vi "EVT Camera Open.vi"(10 "deviceInfo":T1, 11 "cameraHandle":u64) -> (1 "name":string, 2 "deviceInfo out":T1, 3 "cameraHandle out":u64, 4 "function return":u32(ring), 5 "fullName":string)   [LabVIEW 2019, in "EmergentCameraC.lvlib"]
doc: "EMERGENTCAMERAC_API EVT_ERROR EVT_CameraOpen(Camera_Handle* cameraHandle, struct GigEVisionDeviceInfo* deviceInfo);"
uses:
  <vilib>/Utility/importsl/GetValueByPointer/datatype.ctl
  <vilib>/Utility/importsl/GetValueByPointer/GetValueByPointer.xnode
  EmergentCameraC.lvlib
  emergentInstall_Windows/win64/eSDK/bin/EmergentCameraC.dll
types:
  T1 = cluster{"specVersionMajor":u16, "specVersionMinor":u16, "deviceMode":u32, "macAddress[0]":i8, "macAddress[1]":i8, "macAddress[2]":i8, "macAddress[3]":i8, "macAddress[4]":i8, "macAddress[5]":i8, "macAddress[6]":i8, "macAddress[7]":i8, "macAddress[8]":i8, "macAddress[9]":i8, "macAddress[10]":i8, "macAddress[11]":i8, "macAddress[12]":i8, "macAddress[13]":i8, "macAddress[14]":i8, "macAddress[15]":i8, "macAddress[16]":i8, "macAddress[17]":i8, "@dummy control@":i8, "@dummy control@":i8, "ipConfigOptions":u32, "ipConfigCurrent":u32, "currentIp[0]":i8, "currentIp[1]":i8, "currentIp[2]":i8, "currentIp[3]":i8, "currentIp[4]":i8, "currentIp[5]":i8, "currentIp[6]":i8, "currentIp[7]":i8, "currentIp[8]":i8, "currentIp[9]":i8, "currentIp[10]":i8, "currentIp[11]":i8, "currentIp[12]":i8, "currentIp[13]":i8, "currentIp[14]":i8, "currentIp[15]":i8, "currentSubnetMask[0]":i8, "currentSubnetMask[1]":i8, "currentSubnetMask[2]":i8, "currentSubnetMask[3]":i8, "currentSubnetMask[4]":i8, "currentSubnetMask[5]":i8, "currentSubnetMask[6]":i8, "currentSubnetMask[7]":i8, "currentSubnetMask[8]":i8, "currentSubnetMask[9]":i8, "currentSubnetMask[10]":i8, "currentSubnetMask[11]":i8, "currentSubnetMask[12]":i8, "currentSubnetMask[13]":i8, "currentSubnetMask[14]":i8, "currentSubnetMask[15]":i8, "defaultGateway[0]":i8, "defaultGateway[1]":i8, "defaultGateway[2]":i8, "defaultGateway[3]":i8, "defaultGateway[4]":i8, "defaultGateway[5]":i8, "defaultGateway[6]":i8, "defaultGateway[7]":i8, "defaultGateway[8]":i8, "defaultGateway[9]":i8, "defaultGateway[10]":i8, "defaultGateway[11]":i8, "defaultGateway[12]":i8, "defaultGateway[13]":i8, "defaultGateway[14]":i8, "defaultGateway[15]":i8, "manufacturerName[0]":i8, "manufacturerName[1]":i8, "manufacturerName[2]":i8, "manufacturerName[3]":i8, "manufacturerName[4]":i8, "manufacturerName[5]":i8, "manufacturerName[6]":i8, "manufacturerName[7]":i8, "manufacturerName[8]":i8, "manufacturerName[9]":i8, "manufacturerName[10]":i8, "manufacturerName[11]":i8, "manufacturerName[12]":i8, "manufacturerName[13]":i8, "manufacturerName[14]":i8, "manufacturerName[15]":i8, "manufacturerName[16]":i8, "manufacturerName[17]":i8, "manufacturerName[18]":i8, "manufacturerName[19]":i8, "manufacturerName[20]":i8, "manufacturerName[21]":i8, "manufacturerName[22]":i8, "manufacturerName[23]":i8, "manufacturerName[24]":i8, "manufacturerName[25]":i8, "manufacturerName[26]":i8, "manufacturerName[27]":i8, "manufacturerName[28]":i8, "manufacturerName[29]":i8, "manufacturerName[30]":i8, "manufacturerName[31]":i8, "modelName[0]":i8, "modelName[1]":i8, "modelName[2]":i8, "modelName[3]":i8, "modelName[4]":i8, "modelName[5]":i8, "modelName[6]":i8, "modelName[7]":i8, "modelName[8]":i8, "modelName[9]":i8, "modelName[10]":i8, "modelName[11]":i8, "modelName[12]":i8, "modelName[13]":i8, "modelName[14]":i8, "modelName[15]":i8, "modelName[16]":i8, "modelName[17]":i8, "modelName[18]":i8, "modelName[19]":i8, "modelName[20]":i8, "modelName[21]":i8, "modelName[22]":i8, "modelName[23]":i8, "modelName[24]":i8, "modelName[25]":i8, "modelName[26]":i8, "modelName[27]":i8, "modelName[28]":i8, "modelName[29]":i8, "modelName[30]":i8, "modelName[31]":i8, "deviceVersion[0]":i8, "deviceVersion[1]":i8, "deviceVersion[2]":i8, "deviceVersion[3]":i8, "deviceVersion[4]":i8, "deviceVersion[5]":i8, "deviceVersion[6]":i8, "deviceVersion[7]":i8, "deviceVersion[8]":i8, "deviceVersion[9]":i8, "deviceVersion[10]":i8, "deviceVersion[11]":i8, "deviceVersion[12]":i8, "deviceVersion[13]":i8, "deviceVersion[14]":i8, "deviceVersion[15]":i8, "deviceVersion[16]":i8, "deviceVersion[17]":i8, "deviceVersion[18]":i8, "deviceVersion[19]":i8, "deviceVersion[20]":i8, "deviceVersion[21]":i8, "deviceVersion[22]":i8, "deviceVersion[23]":i8, "deviceVersion[24]":i8, "deviceVersion[25]":i8, "deviceVersion[26]":i8, "deviceVersion[27]":i8, "deviceVersion[28]":i8, "deviceVersion[29]":i8, "deviceVersion[30]":i8, "deviceVersion[31]":i8, "manufacturerSpecifiedInfo[0]":i8, "manufacturerSpecifiedInfo[1]":i8, "manufacturerSpecifiedInfo[2]":i8, "manufacturerSpecifiedInfo[3]":i8, "manufacturerSpecifiedInfo[4]":i8, "manufacturerSpecifiedInfo[5]":i8, "manufacturerSpecifiedInfo[6]":i8, "manufacturerSpecifiedInfo[7]":i8, "manufacturerSpecifiedInfo[8]":i8, "manufacturerSpecifiedInfo[9]":i8, "manufacturerSpecifiedInfo[10]":i8, "manufacturerSpecifiedInfo[11]":i8, "manufacturerSpecifiedInfo[12]":i8, "manufacturerSpecifiedInfo[13]":i8, "manufacturerSpecifiedInfo[14]":i8, "manufacturerSpecifiedInfo[15]":i8, "manufacturerSpecifiedInfo[16]":i8, "manufacturerSpecifiedInfo[17]":i8, "manufacturerSpecifiedInfo[18]":i8, "manufacturerSpecifiedInfo[19]":i8, "manufacturerSpecifiedInfo[20]":i8, "manufacturerSpecifiedInfo[21]":i8, "manufacturerSpecifiedInfo[22]":i8, "manufacturerSpecifiedInfo[23]":i8, "manufacturerSpecifiedInfo[24]":i8, "manufacturerSpecifiedInfo[25]":i8, "manufacturerSpecifiedInfo[26]":i8, "manufacturerSpecifiedInfo[27]":i8, "manufacturerSpecifiedInfo[28]":i8, "manufacturerSpecifiedInfo[29]":i8, "manufacturerSpecifiedInfo[30]":i8, "manufacturerSpecifiedInfo[31]":i8, "manufacturerSpecifiedInfo[32]":i8, "manufacturerSpecifiedInfo[33]":i8, "manufacturerSpecifiedInfo[34]":i8, "manufacturerSpecifiedInfo[35]":i8, "manufacturerSpecifiedInfo[36]":i8, "manufacturerSpecifiedInfo[37]":i8, "manufacturerSpecifiedInfo[38]":i8, "manufacturerSpecifiedInfo[39]":i8, "manufacturerSpecifiedInfo[40]":i8, "manufacturerSpecifiedInfo[41]":i8, "manufacturerSpecifiedInfo[42]":i8, "manufacturerSpecifiedInfo[43]":i8, "manufacturerSpecifiedInfo[44]":i8, "manufacturerSpecifiedInfo[45]":i8, "manufacturerSpecifiedInfo[46]":i8, "manufacturerSpecifiedInfo[47]":i8, "serialNumber[0]":i8, "serialNumber[1]":i8, "serialNumber[2]":i8, "serialNumber[3]":i8, "serialNumber[4]":i8, "serialNumber[5]":i8, "serialNumber[6]":i8, "serialNumber[7]":i8, "serialNumber[8]":i8, "serialNumber[9]":i8, "serialNumber[10]":i8, "serialNumber[11]":i8, "serialNumber[12]":i8, "serialNumber[13]":i8, "serialNumber[14]":i8, "serialNumber[15]":i8, "userDefinedName[0]":i8, "userDefinedName[1]":i8, "userDefinedName[2]":i8, "userDefinedName[3]":i8, "userDefinedName[4]":i8, "userDefinedName[5]":i8, "userDefinedName[6]":i8, "userDefinedName[7]":i8, "userDefinedName[8]":i8, "userDefinedName[9]":i8, "userDefinedName[10]":i8, "userDefinedName[11]":i8, "userDefinedName[12]":i8, "userDefinedName[13]":i8, "userDefinedName[14]":i8, "userDefinedName[15]":i8, "ip4Address[0]":i8, "ip4Address[1]":i8, "ip4Address[2]":i8, "ip4Address[3]":i8, "ip4Address[4]":i8, "ip4Address[5]":i8, "ip4Address[6]":i8, "ip4Address[7]":i8, "ip4Address[8]":i8, "ip4Address[9]":i8, "ip4Address[10]":i8, "ip4Address[11]":i8, "ip4Address[12]":i8, "ip4Address[13]":i8, "ip4Address[14]":i8, "ip4Address[15]":i8, "ip4AddressBroadcast[0]":i8, "ip4AddressBroadcast[1]":i8, "ip4AddressBroadcast[2]":i8, "ip4AddressBroadcast[3]":i8, "ip4AddressBroadcast[4]":i8, "ip4AddressBroadcast[5]":i8, "ip4AddressBroadcast[6]":i8, "ip4AddressBroadcast[7]":i8, "ip4AddressBroadcast[8]":i8, "ip4AddressBroadcast[9]":i8, "ip4AddressBroadcast[10]":i8, "ip4AddressBroadcast[11]":i8, "ip4AddressBroadcast[12]":i8, "ip4AddressBroadcast[13]":i8, "ip4AddressBroadcast[14]":i8, "ip4AddressBroadcast[15]":i8, "friendlyName[0]":i8, "friendlyName[1]":i8, "friendlyName[2]":i8, "friendlyName[3]":i8, "friendlyName[4]":i8, "friendlyName[5]":i8, "friendlyName[6]":i8, "friendlyName[7]":i8, "friendlyName[8]":i8, "friendlyName[9]":i8, "friendlyName[10]":i8, "friendlyName[11]":i8, "friendlyName[12]":i8, "friendlyName[13]":i8, "friendlyName[14]":i8, "friendlyName[15]":i8, "friendlyName[16]":i8, "friendlyName[17]":i8, "friendlyName[18]":i8, "friendlyName[19]":i8, "friendlyName[20]":i8, "friendlyName[21]":i8, "friendlyName[22]":i8, "friendlyName[23]":i8, "friendlyName[24]":i8, "friendlyName[25]":i8, "friendlyName[26]":i8, "friendlyName[27]":i8, "friendlyName[28]":i8, "friendlyName[29]":i8, "friendlyName[30]":i8, "friendlyName[31]":i8, "friendlyName[32]":i8, "friendlyName[33]":i8, "friendlyName[34]":i8, "friendlyName[35]":i8, "friendlyName[36]":i8, "friendlyName[37]":i8, "friendlyName[38]":i8, "friendlyName[39]":i8, "friendlyName[40]":i8, "friendlyName[41]":i8, "friendlyName[42]":i8, "friendlyName[43]":i8, "friendlyName[44]":i8, "friendlyName[45]":i8, "friendlyName[46]":i8, "friendlyName[47]":i8, "friendlyName[48]":i8, "friendlyName[49]":i8, "friendlyName[50]":i8, "friendlyName[51]":i8, "friendlyName[52]":i8, "friendlyName[53]":i8, "friendlyName[54]":i8, "friendlyName[55]":i8, "friendlyName[56]":i8, "friendlyName[57]":i8, "friendlyName[58]":i8, "friendlyName[59]":i8, "friendlyName[60]":i8, "friendlyName[61]":i8, "friendlyName[62]":i8, "friendlyName[63]":i8, "friendlyName[64]":i8, "friendlyName[65]":i8, "friendlyName[66]":i8, "friendlyName[67]":i8, "friendlyName[68]":i8, "friendlyName[69]":i8, "friendlyName[70]":i8, "friendlyName[71]":i8, "friendlyName[72]":i8, "friendlyName[73]":i8, "friendlyName[74]":i8, "friendlyName[75]":i8, "friendlyName[76]":i8, "friendlyName[77]":i8, "friendlyName[78]":i8, "friendlyName[79]":i8, "friendlyName[80]":i8, "friendlyName[81]":i8, "friendlyName[82]":i8, "friendlyName[83]":i8, "friendlyName[84]":i8, "friendlyName[85]":i8, "friendlyName[86]":i8, "friendlyName[87]":i8, "friendlyName[88]":i8, "friendlyName[89]":i8, "friendlyName[90]":i8, "friendlyName[91]":i8, "friendlyName[92]":i8, "friendlyName[93]":i8, "friendlyName[94]":i8, "friendlyName[95]":i8, "friendlyName[96]":i8, "friendlyName[97]":i8, "friendlyName[98]":i8, "friendlyName[99]":i8, "friendlyName[100]":i8, "friendlyName[101]":i8, "friendlyName[102]":i8, "friendlyName[103]":i8, "friendlyName[104]":i8, "friendlyName[105]":i8, "friendlyName[106]":i8, "friendlyName[107]":i8, "friendlyName[108]":i8, "friendlyName[109]":i8, "friendlyName[110]":i8, "friendlyName[111]":i8, "friendlyName[112]":i8, "friendlyName[113]":i8, "friendlyName[114]":i8, "friendlyName[115]":i8, "friendlyName[116]":i8, "friendlyName[117]":i8, "friendlyName[118]":i8, "friendlyName[119]":i8, "friendlyName[120]":i8, "friendlyName[121]":i8, "friendlyName[122]":i8, "friendlyName[123]":i8, "friendlyName[124]":i8, "friendlyName[125]":i8, "friendlyName[126]":i8, "friendlyName[127]":i8, "description[0]":i8, "description[1]":i8, "description[2]":i8, "description[3]":i8, "description[4]":i8, "description[5]":i8, "description[6]":i8, "description[7]":i8, "description[8]":i8, "description[9]":i8, "description[10]":i8, "description[11]":i8, "description[12]":i8, "description[13]":i8, "description[14]":i8, "description[15]":i8, "description[16]":i8, "description[17]":i8, "description[18]":i8, "description[19]":i8, "description[20]":i8, "description[21]":i8, "description[22]":i8, "description[23]":i8, "description[24]":i8, "description[25]":i8, "description[26]":i8, "description[27]":i8, "description[28]":i8, "description[29]":i8, "description[30]":i8, "description[31]":i8, "description[32]":i8, "description[33]":i8, "description[34]":i8, "description[35]":i8, "description[36]":i8, "description[37]":i8, "description[38]":i8, "description[39]":i8, "description[40]":i8, "description[41]":i8, "description[42]":i8, "description[43]":i8, "description[44]":i8, "description[45]":i8, "description[46]":i8, "description[47]":i8, "description[48]":i8, "description[49]":i8, "description[50]":i8, "description[51]":i8, "description[52]":i8, "description[53]":i8, "description[54]":i8, "description[55]":i8, "description[56]":i8, "description[57]":i8, "description[58]":i8, "description[59]":i8, "description[60]":i8, "description[61]":i8, "description[62]":i8, "description[63]":i8, "description[64]":i8, "description[65]":i8, "description[66]":i8, "description[67]":i8, "description[68]":i8, "description[69]":i8, "description[70]":i8, "description[71]":i8, "description[72]":i8, "description[73]":i8, "description[74]":i8, "description[75]":i8, "description[76]":i8, "description[77]":i8, "description[78]":i8, "description[79]":i8, "description[80]":i8, "description[81]":i8, "description[82]":i8, "description[83]":i8, "description[84]":i8, "description[85]":i8, "description[86]":i8, "description[87]":i8, "description[88]":i8, "description[89]":i8, "description[90]":i8, "description[91]":i8, "description[92]":i8, "description[93]":i8, "description[94]":i8, "description[95]":i8, "description[96]":i8, "description[97]":i8, "description[98]":i8, "description[99]":i8, "description[100]":i8, "description[101]":i8, "description[102]":i8, "description[103]":i8, "description[104]":i8, "description[105]":i8, "description[106]":i8, "description[107]":i8, "description[108]":i8, "description[109]":i8, "description[110]":i8, "description[111]":i8, "description[112]":i8, "description[113]":i8, "description[114]":i8, "description[115]":i8, "description[116]":i8, "description[117]":i8, "description[118]":i8, "description[119]":i8, "description[120]":i8, "description[121]":i8, "description[122]":i8, "description[123]":i8, "description[124]":i8, "description[125]":i8, "description[126]":i8, "description[127]":i8, "adapterName[0]":i8, "adapterName[1]":i8, "adapterName[2]":i8, "adapterName[3]":i8, "adapterName[4]":i8, "adapterName[5]":i8, "adapterName[6]":i8, "adapterName[7]":i8, "adapterName[8]":i8, "adapterName[9]":i8, "adapterName[10]":i8, "adapterName[11]":i8, "adapterName[12]":i8, "adapterName[13]":i8, "adapterName[14]":i8, "adapterName[15]":i8, "adapterName[16]":i8, "adapterName[17]":i8, "adapterName[18]":i8, "adapterName[19]":i8, "adapterName[20]":i8, "adapterName[21]":i8, "adapterName[22]":i8, "adapterName[23]":i8, "adapterName[24]":i8, "adapterName[25]":i8, "adapterName[26]":i8, "adapterName[27]":i8, "adapterName[28]":i8, "adapterName[29]":i8, "adapterName[30]":i8, "adapterName[31]":i8, "adapterName[32]":i8, "adapterName[33]":i8, "adapterName[34]":i8, "adapterName[35]":i8, "adapterName[36]":i8, "adapterName[37]":i8, "adapterName[38]":i8, "adapterName[39]":i8, "adapterName[40]":i8, "adapterName[41]":i8, "adapterName[42]":i8, "adapterName[43]":i8, "adapterName[44]":i8, "adapterName[45]":i8, "adapterName[46]":i8, "adapterName[47]":i8, "adapterName[48]":i8, "adapterName[49]":i8, "adapterName[50]":i8, "adapterName[51]":i8, "adapterName[52]":i8, "adapterName[53]":i8, "adapterName[54]":i8, "adapterName[55]":i8, "adapterName[56]":i8, "adapterName[57]":i8, "adapterName[58]":i8, "adapterName[59]":i8, "adapterName[60]":i8, "adapterName[61]":i8, "adapterName[62]":i8, "adapterName[63]":i8, "adapterName[64]":i8, "adapterName[65]":i8, "adapterName[66]":i8, "adapterName[67]":i8, "adapterName[68]":i8, "adapterName[69]":i8, "adapterName[70]":i8, "adapterName[71]":i8, "adapterName[72]":i8, "adapterName[73]":i8, "adapterName[74]":i8, "adapterName[75]":i8, "adapterName[76]":i8, "adapterName[77]":i8, "adapterName[78]":i8, "adapterName[79]":i8, "adapterName[80]":i8, "adapterName[81]":i8, "adapterName[82]":i8, "adapterName[83]":i8, "adapterName[84]":i8, "adapterName[85]":i8, "adapterName[86]":i8, "adapterName[87]":i8, "adapterName[88]":i8, "adapterName[89]":i8, "adapterName[90]":i8, "adapterName[91]":i8, "adapterName[92]":i8, "adapterName[93]":i8, "adapterName[94]":i8, "adapterName[95]":i8, "adapterName[96]":i8, "adapterName[97]":i8, "adapterName[98]":i8, "adapterName[99]":i8, "adapterName[100]":i8, "adapterName[101]":i8, "adapterName[102]":i8, "adapterName[103]":i8, "adapterName[104]":i8, "adapterName[105]":i8, "adapterName[106]":i8, "adapterName[107]":i8, "adapterName[108]":i8, "adapterName[109]":i8, "adapterName[110]":i8, "adapterName[111]":i8, "adapterName[112]":i8, "adapterName[113]":i8, "adapterName[114]":i8, "adapterName[115]":i8, "adapterName[116]":i8, "adapterName[117]":i8, "adapterName[118]":i8, "adapterName[119]":i8, "adapterName[120]":i8, "adapterName[121]":i8, "adapterName[122]":i8, "adapterName[123]":i8, "adapterName[124]":i8, "adapterName[125]":i8, "adapterName[126]":i8, "adapterName[127]":i8, "vendorID":u32, "@dummy control@":i8, "@dummy control@":i8, "@dummy control@":i8, "@dummy control@":i8, "@dummy control@":i8, "@dummy control@":i8, "@dummy control@":i8, "@dummy control@":i8, "name":u64, "fullName":u64, "mtu":u32}
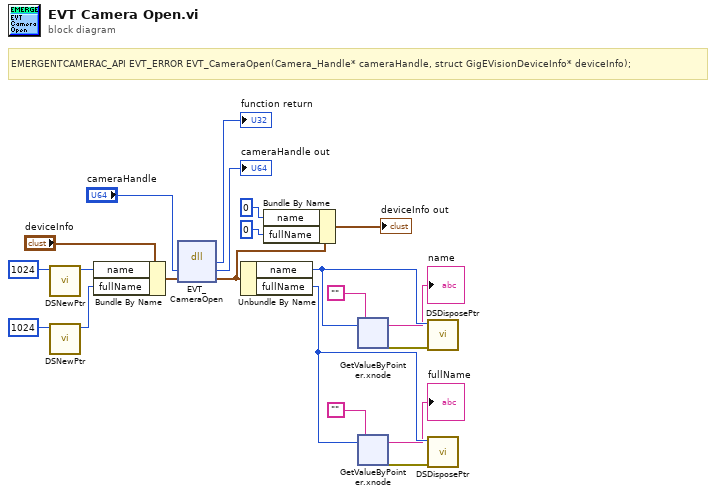
[diagram p0: block diagram]
diagram:
  # "EMERGENTCAMERAC_API EVT_ERROR EVT_CameraOpen(Camera_Handle* cameraHandle, struct GigEVisionDeviceInfo* deviceInfo);"
  n1 = call <vilib>:"DSNewPtr.vi"("Size"=u64 1024) -> ("Pointer"=w15:u64)  [unwired: 9 in, 1 out]
  n2 = call <vilib>:"DSNewPtr.vi"("Size"=u64 1024) -> ("Pointer"=w13:u64)  [unwired: 9 in, 1 out]
  n3 = Bundle By Name(cluster="deviceInfo", "name"=w15, "fullName"=w13) -> (w14:T1)
  n4 = dll-call lib="E:/emergent/host-new_QT/emergentInstall_Windows/win64/eSDK/bin/EmergentCameraC.*" fn="EVT_CameraOpen"("cameraHandle"="cameraHandle", "deviceInfo"=w14) -> (→"function return":u32, "cameraHandle"=→"cameraHandle out":u64, "deviceInfo"=w4:T1)  [unwired: 3 in, 2 out]
  n5 = Unbundle By Name(w4) -> ("name"=w11:u64, "fullName"=w7:u64)
  n6 = Bundle By Name(cluster=w4, "name"=u64 0, "fullName"=u64 0) -> (→"deviceInfo out":T1)
  n7 = xnode "GetValueByPointer.xnode"("Pointer"=w11, "InputType"="") -> ("Output"=→"name":string, "ErrorOut"=w12:errorcluster)  [unwired: 2 in]
  n8 = xnode "GetValueByPointer.xnode"("Pointer"=w7, "InputType"="") -> ("Output"=→"fullName":string, "ErrorOut"=w8:errorcluster)  [unwired: 2 in]
  n9 = call <vilib>:"DSDisposePtr.vi"("error in (no error)"=w12, "Pointer"=w11) -> ()  [unwired: 9 in, 1 out]
  n10 = call <vilib>:"DSDisposePtr.vi"("error in (no error)"=w8, "Pointer"=w7) -> ()  [unwired: 9 in, 1 out]
